vi "To XML - With test suites - Returns aggregated XML.vi"() -> ()   [LabVIEW 2013, in "JUnit XML Tests.lvlib" / "Test Suites.lvlib"]
uses:
  Test Suites.lvlib
  JUnit XML/Test Suite/Test Suite.lvclass/Test Suite.ctl
  JUnit XML/Test Suites/Test Suites.lvclass
  JUnit XML/Test Suite/Write Timestamp.vi
  <vilib>/addons/_JKI Toolkits/Caraya/classes/Assert/Assert Equal Value_Variant.vi
  <vilib>/addons/_JKI Toolkits/Caraya/classes/Test/Test.lvclass
  <vilib>/addons/_JKI Toolkits/Caraya/classes/Assert/Assert.lvclass
  JUnit XML/Test Suite/Test Suite.lvclass
panel:
  out "error out":errorcluster
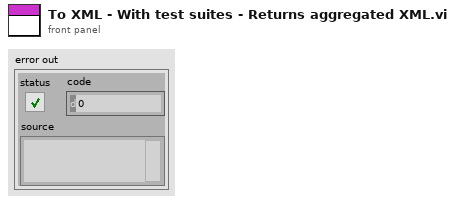
[diagram p1: front panel]
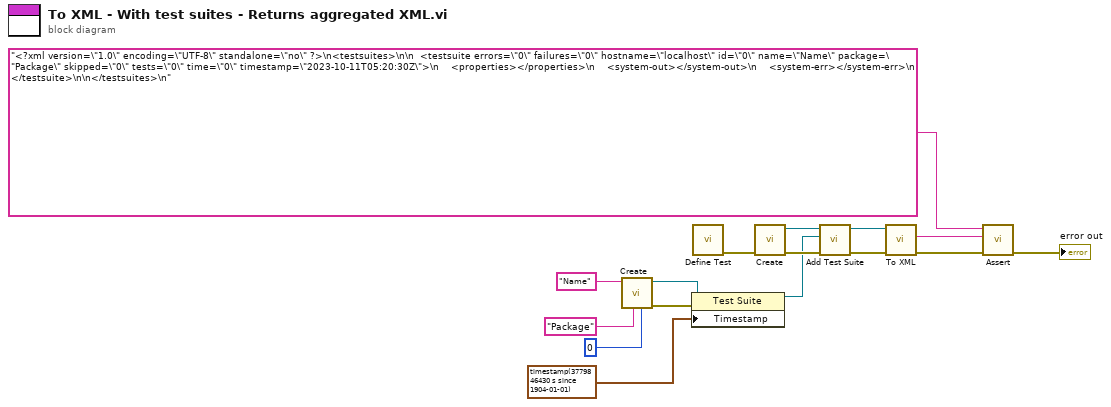
[diagram p0: block diagram]
diagram:
  n1 = call "Create.vi"("Id (-1 = undefined)"=0, "Package (\"\" = undefined)"="Package" ("Package (\"\" = undefined)"), "Name"="Name" ("Package")) -> ("error out"=w10:errorcluster, "Test Suite"=w9:refnum<class "Test Suite.lvclass">)  [unwired: 7 in]
  n2 = property class="Test Suite"(reference=w9, error in=w10, "Timestamp"=timestamp(3779846430.123 s since 1904-01-01)) -> (reference out=w6:refnum<class "Test Suite.lvclass">)  [unwired: 1 out]
  n3 = call <vilib>:"Define Test.vi"() -> ("error out"=w3:errorcluster)  [unwired: 10 in, 1 out]
  n4 = call "Create.vi"("error in (no error)"=w3) -> ("error out"=w14:errorcluster, "Test Suites"=w12:refnum<class "Test Suites.lvclass">)  [unwired: 9 in]
  n5 = call "Add Test Suite.vi"("error in (no error)"=w14, "Test Suite"=w6, "Test Suites in"=w12) -> ("error out"=w13:errorcluster, "Test Suites out"=w11:refnum<class "Test Suites.lvclass">)  [unwired: 7 in]
  n6 = call-dynamic "To XML.vi"("error in (no error)"=w13, "Serializable in"=w11) -> ("error out"=w2:errorcluster, "XML"=w1:string)  [unwired: 8 in]
  n7 = call-poly <vilib>:"Assert.vi"("error in (no error)"=w2, "Actual"=w1, "Expected"="<?xml version=\"1.0\" encoding=\"UTF-8\" standalone=\"no\" ?>\n<testsuites>\n\n  <testsuite errors=\"0\" failures=\"0\" hostname=\"localhost\" id=\"0\" name=\"Name\" package=\"Package\" skipped=\"0\" tests=\"0\" time=\"0\" timestamp=\"2023-10-11T05:20:30Z\">\n    <properties></properties>\n    <system-out></system-out>\n    <system-err></system-err>\n  </testsuite>\n\n</testsuites>\n") -> ("error out"=→"error out":errorcluster)  [unwired: 7 in, 1 out]
